vi "generate graph.vi"(8 "error in (no error)":errorcluster, 9 "waveform slow":waveform(dbl), 10 "waveform fast":waveform(dbl)) -> (0 "error out":errorcluster, 1 "XY Graph 2":cluster{cdb[]}[](graph), 2 "XY Graph":cluster{i32[], "Y":dbl[]}[](graph))   [LabVIEW 2012, in "ImagingModeSPIM.lvclass"]
uses:
  ImagingModeSPIM.lvclass
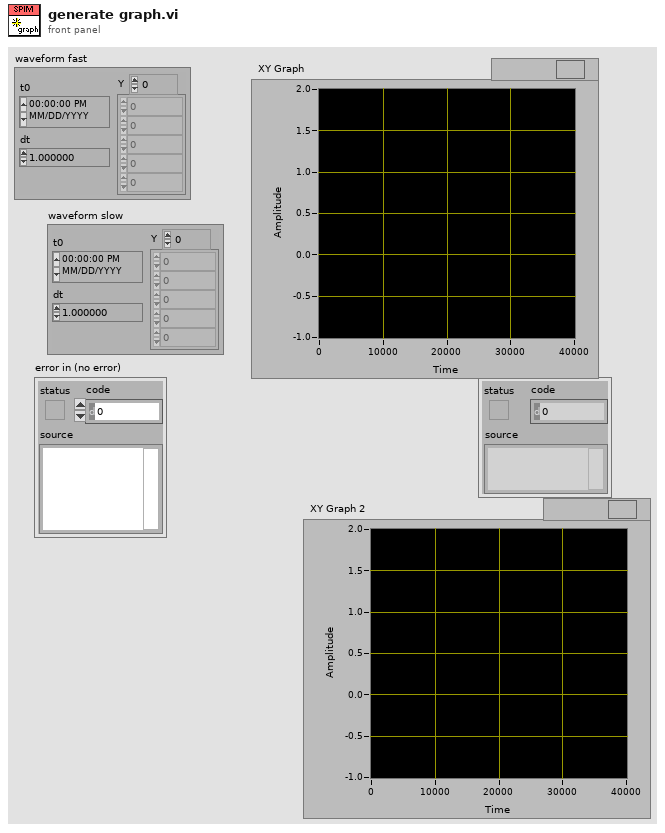
[diagram p1: front panel]
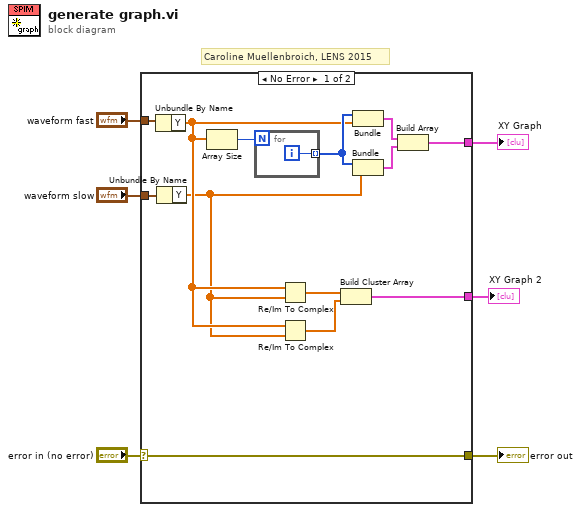
[diagram p0: block diagram]
diagram:
  # "Caroline Muellenbroich, LENS 2015"
  n1 = case shown="No Error" "error in (no error)" {
    selector: "error in (no error)" -> [w19 w21]
    tunnel: [w19 w21] -> w5
    tunnel: "waveform fast" -> [w14 _]
    tunnel: "waveform slow" -> [w13 _]
    tunnel: [w12 _] -> w2
    tunnel: [w7 _] -> w1
    frame No Error {
      n2 = Unbundle By Name(w14) -> ("Y"=w11:dbl[])
      n3 = Unbundle By Name(w13) -> ("Y"=w10:dbl[])
      n4 = Array Size(array=w11) -> (size(s)=w18:i32)
      n5 = for {
        N: w18 -> [_]
        tunnel: [w20] -> w15 mode=indexing
        i -> [w20]
      }
      n6 = Re/Im To Complex(1:w10, 2:w11) -> (0:w9:cdb[])
      n7 = Re/Im To Complex(1:w10, 2:w11) -> (0:w8:cdb[])
      n8 = Build Cluster Array(w9, w8) -> (w7:cluster{cdb[]}[])
      n9 = Bundle(w15, "Y"=w11) -> (w16:cluster{i32[], "Y":dbl[]})  [unwired: 1 in]
      n10 = Bundle(w15, "Y"=w10) -> (w17:cluster{i32[], "Y":dbl[]})  [unwired: 1 in]
      n11 = Build Array(w16, w17) -> (w12:cluster{i32[], "Y":dbl[]}[])
    }
    frame Error {
    }
  }
  "error out" <- w5
  "XY Graph" <- w2
  "XY Graph 2" <- w1
